vi "LogitechF310_JoyStick_map - Copy.vi"(3 "JoystickDevRef":T3) -> (0 "ButtonsCluster":T1, 1 "POVCluster":cluster{i16, i16, i16, i16, i16, i16, i16, i16}, 2 "AxesCluster":T2)   [LabVIEW 2015]
uses:
  <vilib>/Rock Robotics/Network Tables/SD Write Boolean Array.vi
  <vilib>/Rock Robotics/Network Tables/SD Write Numeric Array.vi
  <vilib>/Rock Robotics/WPI/Joystick/WPI_JoystickDeviceEnum.ctl
  <vilib>/Rock Robotics/WPI/Joystick/WPI_JoystickDevRef.ctl
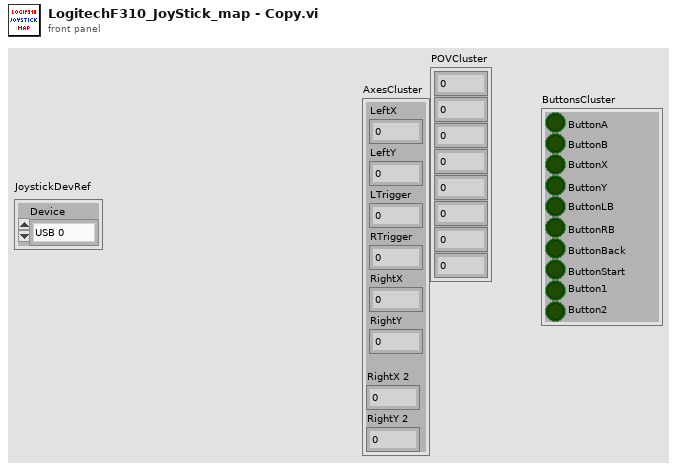
[diagram p1: front panel]
types:
  T1 = cluster{"ButtonA":bool, "ButtonB":bool, "ButtonX":bool, "ButtonY":bool, "ButtonLB":bool, "ButtonRB":bool, "ButtonBack":bool, "ButtonStart":bool, "Button1":bool, "Button2":bool}
  T2 = cluster{"LeftX":dbl, "LeftY":dbl, "LTrigger":dbl, "RTrigger":dbl, "RightX":dbl, "RightY":dbl, "RightY 2":dbl, "RightX 2":dbl}
  T3 = typedef "WPI_JoystickDevRef.ctl" = cluster{"Device":T4}
  T4 = typedef "WPI_JoystickDeviceEnum.ctl" = enum16{"USB 0", "USB 1", "USB 2", "USB 3", "USB 4", "USB 5"}
  T5 = cluster{"upper limit":dbl, "upper limit":dbl, "upper limit":dbl, "upper limit":dbl, "upper limit":dbl, "upper limit":dbl, "upper limit":dbl, "upper limit":dbl}
  T6 = cluster{i16, i16, i16, i16, i16, i16, i16, i16, i16}
  T7 = cluster{bool, bool, bool, bool, bool, bool, bool, bool, bool, bool}
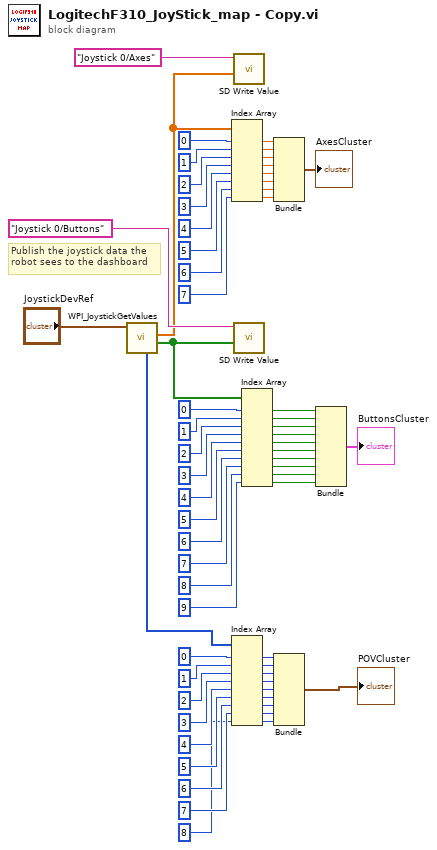
[diagram p0: block diagram]
diagram:
  # "Publish the joystick data the\nrobot sees to the dashboard"
  n1 = call <vilib>:"WPI_JoystickGetValues.vi"("JoystickDevRef"="JoystickDevRef") -> ("Buttons"=w57:bool[], "Axes"=w62:dbl[], "POVs"=w20:i16[])  [unwired: 6 in, 2 out]
  n2 = Index Array(array=w62, index #1=0, index #2=1, index #3=2 ("index"), index #4=3 ("index"), index #5=4 ("index"), index #6=5 ("index"), index #7=6, index #8=7) -> (element #1=w44:dbl, element #2=w43:dbl, element #3=w42:dbl, element #4=w41:dbl, element #5=w38:dbl, element #6=w37:dbl, element #7=w22:dbl, element #8=w21:dbl)
  n3 = Index Array(array=w20, index #1=0 ("index"), index #2=1 ("index"), index #3=2 ("index"), index #4=3 ("index"), index #5=4 ("index"), index #6=5 ("index"), index #7=6 ("index"), index #8=7 ("index"), index #9=8 ("index")) -> (element #1=w11:i16, element #2=w10:i16, element #3=w9:i16, element #4=w8:i16, element #5=w7:i16, element #6=w6:i16, element #7=w5:i16, element #8=w4:i16, element #9=w1:i16)
  n4 = call-poly <vilib>:"SD Write Value.vi"("Numeric Array"=w62, "Name"="Joystick 0/Axes") -> ()  [unwired: 8 in, 2 out]
  n5 = call-poly <vilib>:"SD Write Value.vi"("Boolean Array"=w57, "Name"="Joystick 0/Buttons") -> ()  [unwired: 8 in, 2 out]
  n6 = Index Array(array=w57, index #1=0, index #2=1, index #3=2 ("index"), index #4=3 ("index"), index #5=4 ("index"), index #6=5 ("index"), index #7=6 ("index"), index #8=7 ("index"), index #9=8 ("index"), index #10=9 ("index")) -> (element #1=w35:bool, element #2=w34:bool, element #3=w33:bool, element #4=w32:bool, element #5=w31:bool, element #6=w30:bool, element #7=w29:bool, element #8=w28:bool, element #9=w27:bool, element #10=w26:bool)
  n7 = Bundle("upper limit"=w44, "upper limit"=w43, "upper limit"=w42, "upper limit"=w41, "upper limit"=w38, "upper limit"=w37, "upper limit"=w22, "upper limit"=w21) -> (→"AxesCluster":T5)  [unwired: 1 in]
  n8 = Bundle(w11, w10, w9, w8, w7, w6, w5, w4, w1) -> (→"POVCluster":T6)  [unwired: 1 in]
  n9 = Bundle(w35, w34, w33, w32, w31, w30, w29, w28, w27, w26) -> (→"ButtonsCluster":T7)  [unwired: 1 in]
